vi "setTitle.vi"(8 "error in":errorcluster, 11 "fileName":string) -> (0 "error out":errorcluster)   [LabVIEW 2020, in "main.lvlib"]
uses:
  main.lvlib
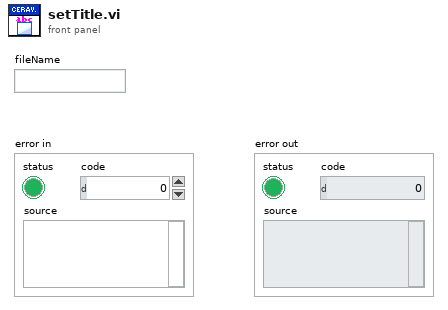
[diagram p1: front panel]
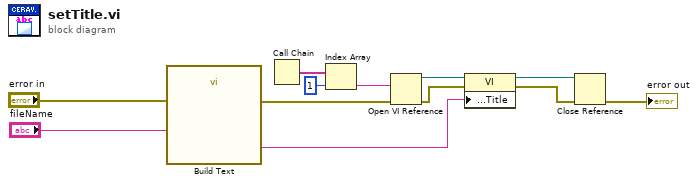
[diagram p0: block diagram]
diagram:
  n1 = call "Build Text"("fileName"="fileName", "error in (no error)"="error in") -> ("Result"=w6:string, "error out"=w5:errorcluster)  [unwired: 12 in]
  n2 = Call Chain() -> (call chain=w12:string[])
  n3 = Index Array(array=w12, index=1) -> (element=w11:string)
  n4 = Open VI Reference(vi path=w11, error in (no error)=w5) -> (vi reference=w10:refnum<vi>, error out=w9:errorcluster)  [unwired: 4 in]
  n5 = property class="VI"(reference=w10, error in=w9, "Front Panel.Title"=w6) -> (reference out=w8:refnum<vi>, error out=w7:errorcluster)
  n6 = Close Reference(reference=w8, error in (no error)=w7) -> (error out=→"error out":errorcluster)
